vi "Lookup Value.vi"(10 "named value":T1, 11 "Nested Actor in":refnum<class "Nested.lvclass">) -> (3 "Nested Actor out":refnum<class "Nested.lvclass">)   [LabVIEW 2023, in "Nested.lvlib" / "Nested.lvclass"]
uses:
  Nested.lvclass
  c:/dev/_r/4/eng/lv-core/lvpostprocessingd/lv_mc_x86_64/dist_i386/vi.lib/ActorFramework/Actor/Actor.lvclass
  Named Value.ctl
  <vilib>/ActorFramework/Actor/Actor.lvclass/Actor.ctl
  Abstraction/Abstraction Messages/Receive Value Msg/Receive Value Msg.lvclass/Receive Value Msg.ctl
  <vilib>/ActorFramework/Message Enqueuer/Message Enqueuer.lvclass/Message Enqueuer.ctl
  <vilib>/ActorFramework/Message Enqueuer/Enqueue.vi
  Abstraction/Abstraction Messages/Receive Value Msg/Receive Value Msg.lvclass
  c:/dev/_r/4/eng/lv-core/lvpostprocessingd/lv_mc_x86_64/dist_i386/vi.lib/ActorFramework/Message/Message.lvclass
  <vilib>/ActorFramework/Message Priority Queue/Priority Enqueue.vi
  <vilib>/ActorFramework/Actor/Actor.lvclass
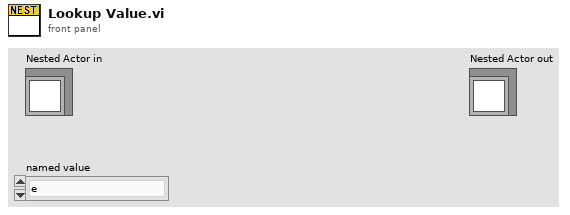
[diagram p1: front panel]
types:
  T1 = typedef "Nested.lvlib/Nested.lvclass/Named Value.ctl" = enum16{"e", "pi", "golden ratio"}
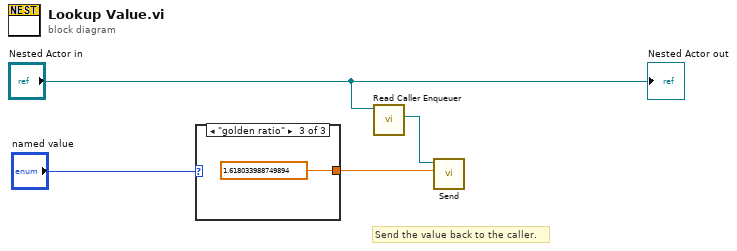
[diagram p0: block diagram]
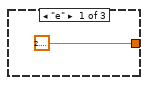
[diagram p2: hidden frame]
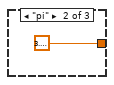
[diagram p3: hidden frame]
diagram:
  # "Send the value back to the caller."
  n1 = case shown="\"golden ratio\"" "named value" {
    tunnel: [2.718281828459045 3.141592653589793 1.618033988749894] -> w3
    frame "e" {
    }
    frame "pi" {
    }
    frame "golden ratio" {
    }
  }
  n2 = call <vilib>:"Read Caller Enqueuer.vi"("Actor"="Nested Actor in") -> ("Caller Enqueuer"=w1:refnum<class "Message Enqueuer.lvclass">)  [unwired: 10 in]
  n3 = call "Send.vi"("Numeric"=w3, "Message Enqueuer"=w1) -> ()  [unwired: 8 in, 2 out]
  "Nested Actor out" <- "Nested Actor in"
